vi "Path Get LF2R Path.vi"(8 "error in (no error)":errorcluster) -> (0 "error out":errorcluster, 2 "Found":bool, 3 "Path":T1)   [LabVIEW 2018, in "Main Panel.lvlib" / "Main Panel.lvclass"]
uses:
  Main Panel.lvclass
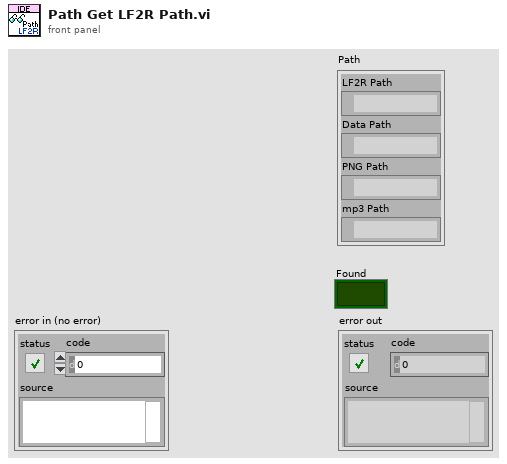
[diagram p1: front panel]
types:
  T1 = cluster{"LF2R Path":path, "Data Path":path, "PNG Path":path, "mp3 Path":path}
  T2 = cluster{"appended path":path, "appended path":path, "appended path":path, "appended path":path}
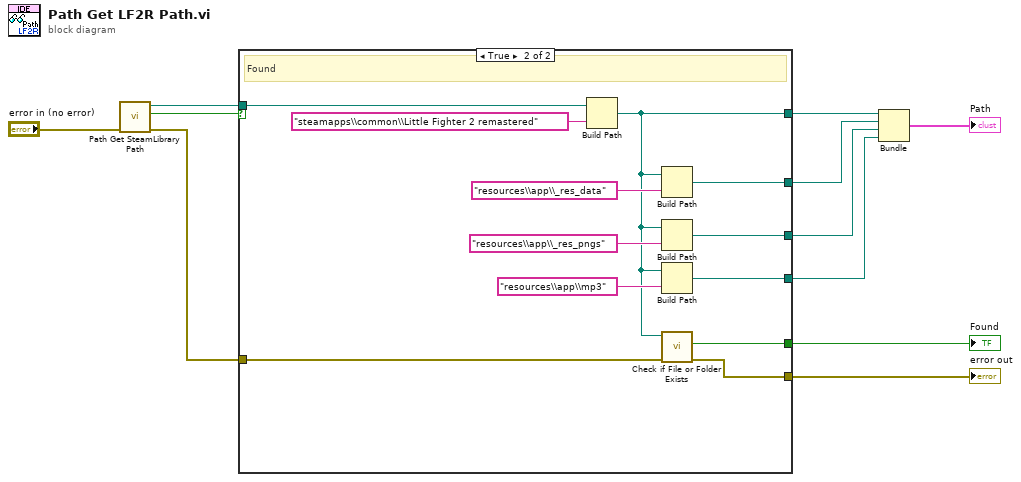
[diagram p0: block diagram]
diagram:
  n1 = call "Path Get SteamLibrary Path.vi"("error in (no error)"="error in (no error)") -> ("error out"=w7:errorcluster, "Found"=w6:bool, "SteamLibrary Path"=w11:path)  [unwired: 8 in]
  n2 = case shown="True" w6 {
    tunnel: w11 -> [_ w24]
    tunnel: [_ w20] -> w3
    tunnel: [_ w19] -> w4
    tunnel: [_ w14] -> w5
    tunnel: [_ w18] -> w9
    tunnel: [w12 w17] -> w8
    tunnel: w7 -> [w12 w16]
    tunnel: [_ w13] -> w2
    frame False {
      # "Not found"
    }
    frame True {
      # "Found"
      n3 = Build Path(base path=w24, name or relative path="steamapps\\common\\Little Fighter 2 remastered") -> (appended path=w14:path)
      n4 = Build Path(base path=w14, name or relative path="resources\\app\\_res_data") -> (appended path=w19:path)
      n5 = Build Path(base path=w14, name or relative path="resources\\app\\_res_pngs") -> (appended path=w20:path)
      n6 = Build Path(base path=w14, name or relative path="resources\\app\\mp3") -> (appended path=w13:path)
      n7 = call <vilib>:"Check if File or Folder Exists.vi"("error in (no error)"=w16, "path"=w14) -> ("error out"=w17:errorcluster, "file or folder exists?"=w18:bool)  [unwired: 7 in, 1 out]
    }
  }
  "error out" <- w8
  "Found" <- w9
  n8 = Bundle("appended path"=w5, "appended path"=w4, "appended path"=w3, "appended path"=w2) -> (→"Path":T2)  [unwired: 1 in]
